vi "run_chatcompletion.vi"(0 "llm_anthropic_chatmodels in":refnum<class "llm_anthropic_chatmodels.lvclass">, 5 "Messages":refnum<class "abstract_message_base.lvclass">[](array[class]), 11 "error in (no error)":errorcluster) -> (4 "llm_anthropic_chatmodels out":refnum<class "llm_anthropic_chatmodels.lvclass">, 6 "Response":refnum<class "abstract_message_base.lvclass">, 15 "error out":errorcluster)   [LabVIEW 2020, in "llm_anthropic_chatmodels.lvclass"]
uses:
  llm_anthropic_chatmodels.lvclass
  abstract_message_base/abstract_message_base.lvclass
  message_text/message_text.lvclass
  D:/Personal/LabVIEW LLMs/src/models/abstract_message_base/abstract_message_base.lvclass
  message_text/message.ctl
  llm_anthropic_chatmodels.lvclass/llm_anthropic_chatmodels.ctl
  <vilib>/httpClient/POSTBuffer.vi
  <vilib>/httpClient/LabVIEWHTTPClient.lvlib
panel:
  out "body":string
  out "headers":string
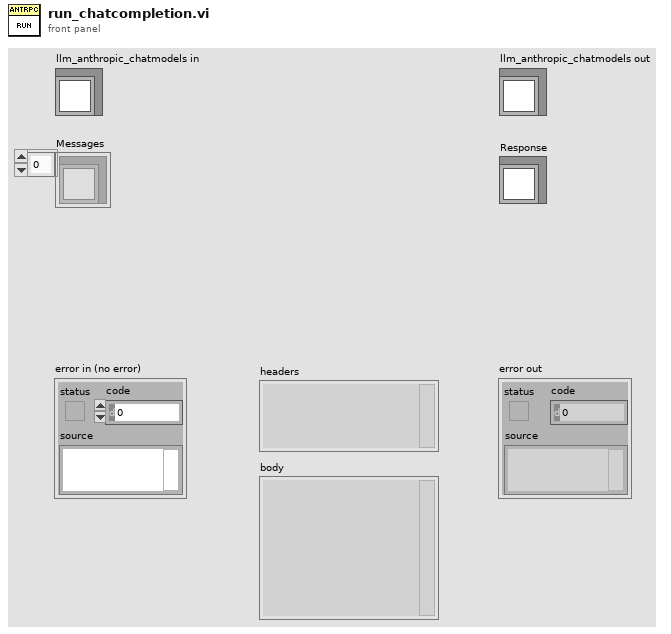
[diagram p1: front panel]
types:
  T1 = typedef "message_text.lvclass/message.ctl" = cluster{"role":string, "content":string[]}
  T2 = typedef "LabVIEWHTTPClient.lvlib/ClientHandle.ctl" = refnum<k1>
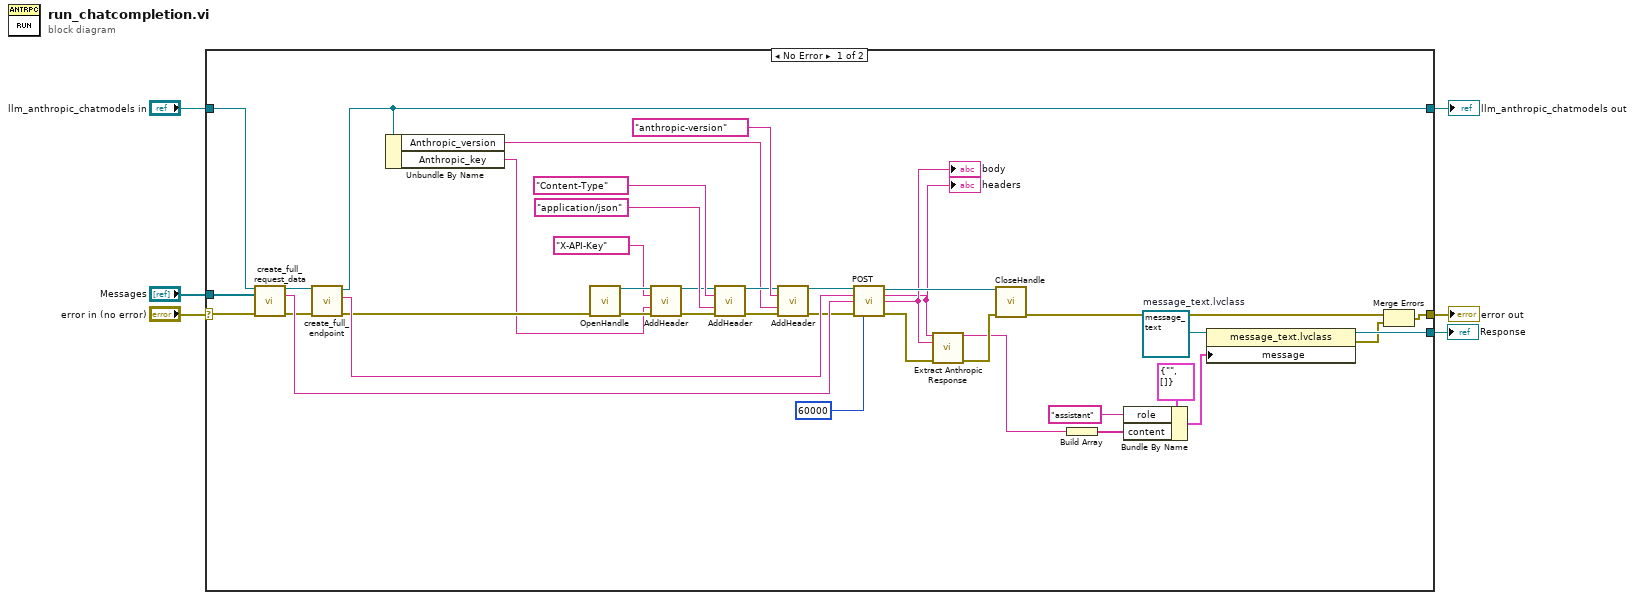
[diagram p0: block diagram]
diagram:
  n1 = case shown="No Error" "error in (no error)" {
    selector: "error in (no error)" -> [w30 w47]
    tunnel: [w33 w47] -> w5
    tunnel: "llm_anthropic_chatmodels in" -> [w32 w46]
    tunnel: [w14 w46] -> w3
    tunnel: "Messages" -> [w31 _]
    tunnel: [w18 _] -> w1
    frame No Error {
      w24 = refnum<class "message_text.lvclass"> refnum  # message_text.lvclass
      n2 = call-dynamic "create_full_request_data.vi"("llm_anthropic_chatmodels in"=w32, "Messages"=w31, "error in (no error)"=w30) -> ("llm_anthropic_chatmodels out"=w28:refnum<class "llm_anthropic_chatmodels.lvclass">, "Request Data"=w29:string, "error out"=w27:errorcluster)  [unwired: 10 in]
      n3 = call-dynamic "create_full_endpoint.vi"("error in (no error)"=w27, "llm_anthropic_chatmodels in"=w28) -> ("error out"=w15:errorcluster, "endpoint"=w26:string, "llm_anthropic_chatmodels out"=w14:refnum<class "llm_anthropic_chatmodels.lvclass">)  [unwired: 7 in]
      n4 = Unbundle By Name(w14) -> ("Anthropic_version"=w7:string, "Anthropic_key"=w8:string)
      n5 = call <vilib>:"OpenHandle.vi"("error in (no error)"=w15) -> ("client handle out"=w45:T2, "error out"=w44:errorcluster)  [unwired: 13 in]
      n6 = call <vilib>:"AddHeader.vi"("client handle"=w45, "header"="X-API-Key", "value"=w8, "error in (no error)"=w44) -> ("client handle out"=w41:T2, "error out"=w40:errorcluster)  [unwired: 10 in]
      n7 = call <vilib>:"AddHeader.vi"("client handle"=w41, "header"="Content-Type", "value"="application/json", "error in (no error)"=w40) -> ("client handle out"=w10:T2, "error out"=w12:errorcluster)  [unwired: 10 in]
      n8 = call <vilib>:"AddHeader.vi"("client handle"=w10, "header"="anthropic-version", "value"=w7, "error in (no error)"=w12) -> ("client handle out"=w9:T2, "error out"=w11:errorcluster)  [unwired: 10 in]
      n9 = call-poly <vilib>:"POST.vi"("client handle"=w9, "url"=w26, "buffer"=w29, "error in (no error)"=w11, "timeout (10000)"=60000) -> ("client handle out"=w38:T2, "headers"=w34:string, "body"=w35:string, "error out"=w37:errorcluster)  [unwired: 7 in]
      "headers" <- w34
      "body" <- w35
      n10 = call "Extract Anthropic Response.vi"("headers"=w34, "body"=w35, "error in"=w37) -> ("value"=w20:string, "error out"=w36:errorcluster)  [unwired: 11 in]
      n11 = call <vilib>:"CloseHandle.vi"("client handle"=w38, "error in (no error)"=w36) -> ("error out"=w39:errorcluster)  [unwired: 13 in]
      n12 = Build Array(w20) -> (w21:string[])
      n13 = Bundle By Name(cluster=T1 {"role"="", "content"=[]} ("message"), "role"="assistant", "content"=w21) -> (w19:T1)
      n14 = property class="message_text.lvclass"(reference=w24, "message"=w19) -> (reference out=w18:refnum<class "message_text.lvclass">, error out=w17:errorcluster)  [unwired: 1 in]
      n15 = Merge Errors(w39, w17) -> (w33:errorcluster)
    }
    frame Error {
    }
  }
  "error out" <- w5
  "llm_anthropic_chatmodels out" <- w3
  "Response" <- w1
